vi "Create Event.vi"(9 "Event":refnum<class "Event.lvclass">, 10 "Self Event Alias":string, 11 "qqqqq in":refnum<class "qqqqq.lvclass">) -> (3 "qqqqq out":refnum<class "qqqqq.lvclass">)   [LabVIEW 2021, in "jettl Tools.lvlib" / "qqqqq.lvlib" / "qqqqq.lvclass"]
uses:
  qqqqq.lvclass
  jettl/Event/Event.lvclass
  qqqqq.lvclass/qqqqq.ctl
  jettl/Queue/Queue.lvclass
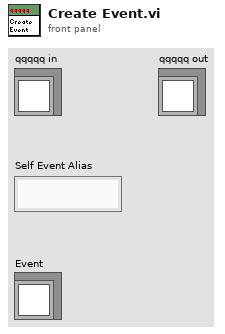
[diagram p1: front panel]
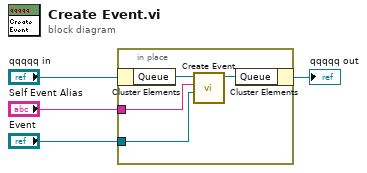
[diagram p0: block diagram]
diagram:
  n1 = in-place {
    in-place-border: "Self Event Alias" -> [w6]
    in-place-border: "Event" -> [w5]
    n2 = in-place-cluster #1("qqqqq in") -> ("Queue"=w8:refnum<class "Queue.lvclass">)
    n3 = call-dynamic "Create Event.vi"("Event"=w5, "Self Event Alias"=w6, "Create Event in"=w8) -> ("Create Event out"=w7:refnum<class "Queue.lvclass">)  [unwired: 8 in]
    n4 = in-place-cluster #1("Queue"=w7) -> (→"qqqqq out":refnum<class "qqqqq.lvclass">)
  }
